vi "Laplacian Convolution.vi"(8 "error in (no error)":errorcluster, 11 "Refnum in":T1) -> (0 "error out":errorcluster, 1 "Mean Value":sgl, 2 "Maximal Value":sgl, 3 "Refnum out":T1, 4 "Standard  Variation":sgl, 5 "Minimal Value":sgl)   [LabVIEW 2016]
uses:
  <vilib>/vision/Image Controls.llb/IMAQ Image.ctl
  <vilib>/vision/NI_Vision_Development_Module.lvlib
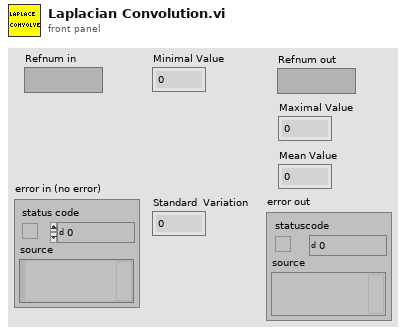
[diagram p1: front panel]
types:
  T1 = typedef "IMAQ Image.ctl" = refnum<image>
  T2 = cluster{"histogram":u32[], "Minimal Value":sgl, "Maximal Value":sgl, "Starting Value":sgl, "Interval Width":sgl, "Mean Value":sgl, "Standard  Variation":sgl, "Area (pixels)":i32}
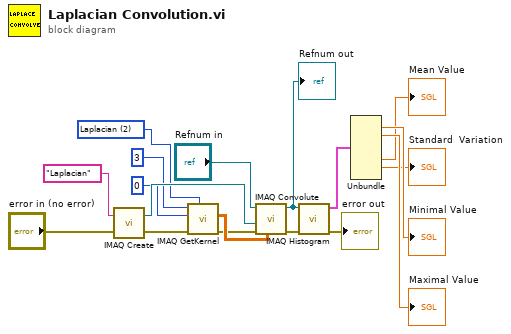
[diagram p0: block diagram]
diagram:
  w9 = u16 2 items=["Gradient"=1, "Laplacian"=2, "Smoothing"=3, "Gaussian"=4] ("Kernel Family")
  n1 = call "IMAQ Create"("Image Name"="Laplacian", "error in (no error)"="error in (no error)") -> ("New Image"=w14:T1, "error out"=w4:errorcluster)  [unwired: 3 in]
  n2 = call "IMAQ GetKernel"("Kernel Family"=w9, "error in (no error)"=w4, "Kernel Number"=0, "Kernel Size (3,5,...)"=3) -> ("error out"=w3:errorcluster, "Kernel"=w16:sgl[][])  [unwired: 4 in, 2 out]
  n3 = call "IMAQ Convolute"("Kernel"=w16, "error in (no error)"=w3, "Image Dst"=w14, "Image Src"="Refnum in") -> ("error out"=w2:errorcluster, "Image Dst Out"=w12:T1)  [unwired: 6 in]
  "Refnum out" <- w12
  n4 = call "IMAQ Histogram"("error in (no error)"=w2, "Image"=w12) -> ("error out"=→"error out":errorcluster, "Histogram Report"=w15:T2)  [unwired: 8 in]
  n5 = Unbundle(w15) -> ("Minimal Value"=→"Minimal Value":sgl, "Maximal Value"=→"Maximal Value":sgl, "Mean Value"=→"Mean Value":sgl, "Standard  Variation"=→"Standard  Variation":sgl)  [unwired: 4 out]
